vi "Initiate Trigger System.vi"(8 "error in (no error)":errorcluster, 9 "Operation (0 : Initiate Trigger Once)":u16(ring) items=["Initiate Trigger Once", "Initiate Trigger Continuously", "Stop Continuously Trigger"], 10 "Channel (1)":string="1", 11 "VISA resource name":refnum<visa-resource-name>) -> (0 "error out":errorcluster, 3 "VISA resource name out":refnum<visa-resource-name>)   [LabVIEW 2020, in "Keysight E36300 Series.lvlib"]
doc: "Initiates the output trigger system."
uses:
  Keysight E36300 Series.lvlib
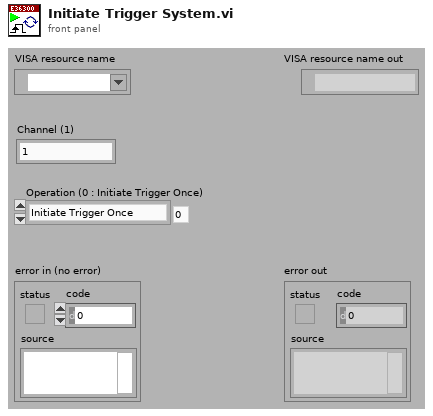
[diagram p1: front panel]
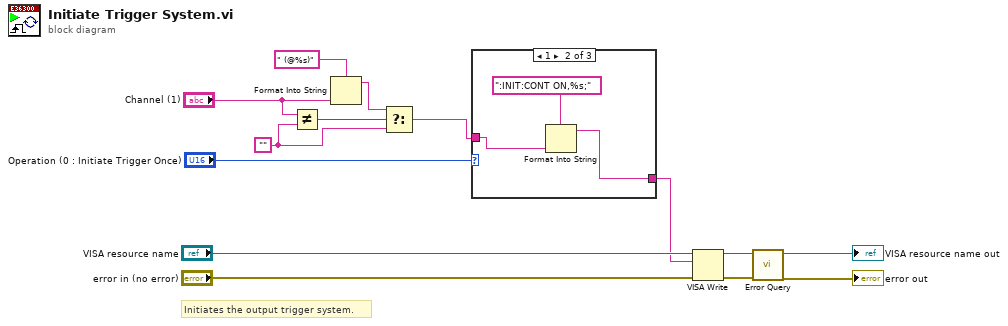
[diagram p0: block diagram]
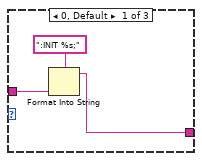
[diagram p2: hidden frame]
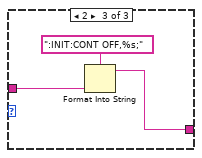
[diagram p3: hidden frame]
diagram:
  w1 = ""
  # "Initiates the output trigger system."
  n1 = Not Equal?(x="Channel (1)", y=w1) -> (x != y?=w4:bool)
  n2 = Format Into String(format string=" (@%s)", "Channel (1)") -> (resulting string=w5:string)  [unwired: 2 in, 1 out]
  n3 = Select(t=w5, s=w4, f=w1) -> (s? t:f=w2:string)
  n4 = case shown="1" "Operation (0 : Initiate Trigger Once)" {
    tunnel: [w17 w20 w22] -> w8
    tunnel: w2 -> [w15 w18 w21]
    frame 0, Default {
      n5 = Format Into String(format string=":INIT %s;", w15) -> (resulting string=w17:string)  [unwired: 2 in, 1 out]
    }
    frame 1 {
      n6 = Format Into String(format string=":INIT:CONT ON,%s;", w18) -> (resulting string=w20:string)  [unwired: 2 in, 1 out]
    }
    frame 2 {
      n7 = Format Into String(format string=":INIT:CONT OFF,%s;", w21) -> (resulting string=w22:string)  [unwired: 2 in, 1 out]
    }
  }
  n8 = VISA Write(VISA resource name="VISA resource name", write buffer=w8, error in (no error)="error in (no error)") -> (VISA resource name out=w12:refnum<visa-resource-name>, error out=w11:errorcluster)  [unwired: 1 out]
  n9 = call "Error Query.vi"("error in (no error)"=w11, "VISA resource name"=w12) -> ("error out"=→"error out":errorcluster, "VISA resource name out"=→"VISA resource name out":refnum<visa-resource-name>)  [unwired: 6 in, 2 out]
